vi "lsl prepend child value.vi"(8 "error in (no error)":errorcluster, 9 "value":string, 10 "name":string, 11 "xml_ptr":T1) -> (0 "error out":errorcluster, 2 "function return":u32, 3 "xml_ptr out":T1)   [LabVIEW 2016, in "Lab Streaming Layer.lvlib"]
doc: "extern LIBLSL_C_API lsl_xml_ptr lsl_prepend_child_value(lsl_xml_ptr e, const char *name, const char *value);"
uses:
  Lab Streaming Layer.lvlib
  liblsl-LabVIEW-master/liblsl-LabVIEW-master/lsl.dll
  Custom Controls/lsl_xml_ptr.ctl
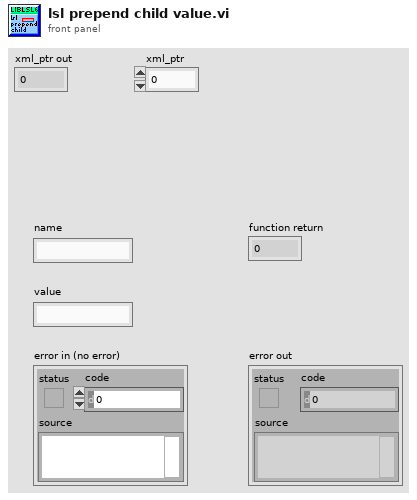
[diagram p1: front panel]
types:
  T1 = typedef "liblsl-LabVIEW.lvlib/lsl_xml_ptr.ctl" = u64
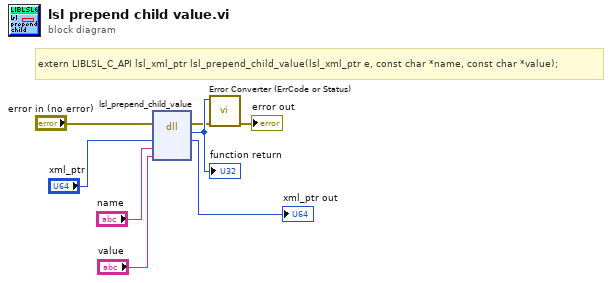
[diagram p0: block diagram]
diagram:
  # "extern LIBLSL_C_API lsl_xml_ptr lsl_prepend_child_value(lsl_xml_ptr e, const char *name, const char *value);"
  n1 = dll-call lib="E:/LabStreamingLayer/liblsl-LabVIEW-master/liblsl-LabVIEW-master/lsl.dll" fn="lsl_prepend_child_value"(error in="error in (no error)", "xml_ptr"="xml_ptr", "name"="name", "value"="value") -> (error out=w4:errorcluster, "return type"=w8:u32, "xml_ptr"=→"xml_ptr out":u64)  [unwired: 4 in, 1 out]
  "function return" <- w8
  n2 = call "Error Converter (ErrCode or Status).vi"("error in (no error)"=w4, "error code"=w8) -> ("error out"=→"error out":errorcluster)  [unwired: 9 in]
